vi "Debug Get Connected Units.vi"() -> ()   [LabVIEW 2021]
uses:
  <vilib>/Utility/config.llb/NI_LVConfig.lvlib
  <vilib>/Utility/config.llb/Read Key (Boolean).vi
panel:
  out "Array":T1(array[cluster])
  in  "stop":bool
  in  "UDP Config Publish Port":u16
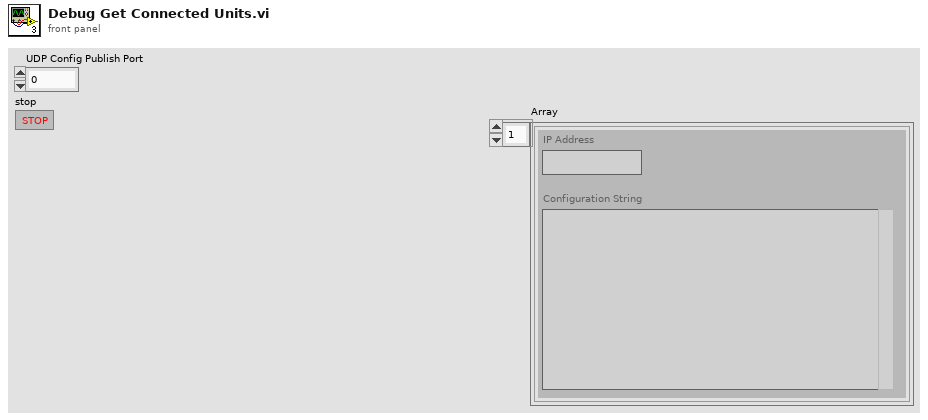
[diagram p1: front panel]
types:
  T1 = cluster{"IP Address":string, "Configuration String":string}[]
  T2 = cluster{"IP Address":string, "Configuration String":string}
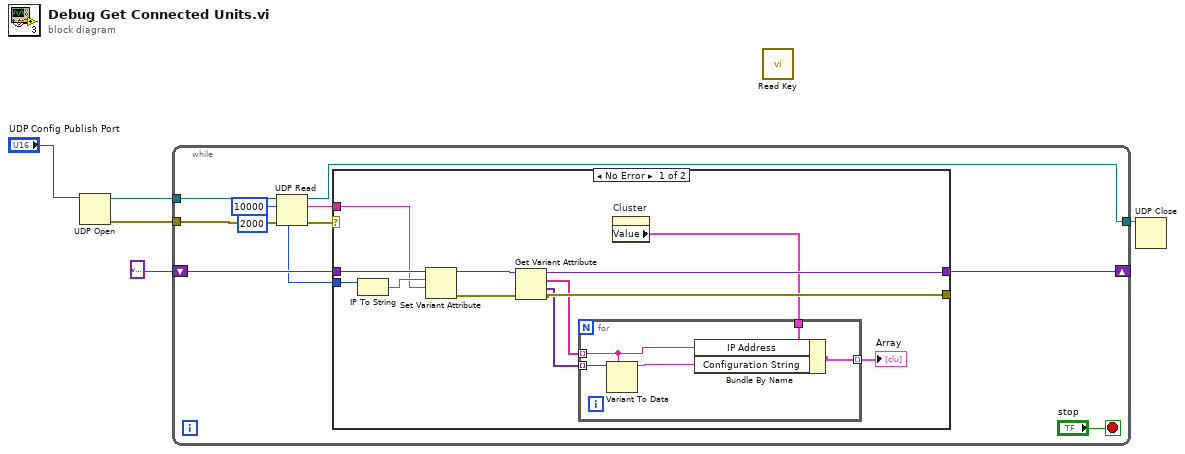
[diagram p0: block diagram]
diagram:
  n1 = UDP Open(11:"UDP Config Publish Port") -> (port=w3:refnum<k16>, 0:w4:errorcluster)  [unwired: 4 in, 1 out]
  n2 = while {
    tunnel: w4 -> [w16]
    tunnel: w3 -> [w15]
    shift-right: [w9] -> _
    shift-left: variant -> [w13]
    tunnel: [w7] -> w1
    stop <- "stop" stop-if-true
    n3 = UDP Read(connection ID=w15, max size (548)=10000, timeout ms (25000)=2000, 8:w16) -> (data out=w12:string, error out=w11:errorcluster, 3:w7:refnum<k16>, 6:w6:u32)  [unwired: 1 out]
    n4 = case shown="No Error" w11 {
      tunnel: w13 -> [w28 w34]
      tunnel: w6 -> [w26 _]
      tunnel: w12 -> [w25 _]
      tunnel: [w23 w34] -> w9
      tunnel: [w21 _] -> _
      frame No Error {
        n5 = IP To String(2:w26) -> (0:w27:string)  [unwired: 1 in]
        n6 = Set Variant Attribute(Variant=w28, name=w27, value=w25) -> (Variant out=w24:variant, error out=w22:errorcluster)  [unwired: 1 in, 1 out]
        n7 = Get Variant Attribute(Variant=w24, error in=w22) -> (duplicate Variant=w23:variant, names=w20:string[], values=w19:variant[], error out=w21:errorcluster)  [unwired: 2 in]
        n8 = property on="Cluster" class="Clust (strict)"() -> ("Value"=w18:T2)  [unwired: 2 in, 2 out]
        n9 = for {
          tunnel: w20 -> [w31] mode=indexing
          tunnel: w19 -> [w33] mode=indexing
          tunnel: w18 -> [w32]
          tunnel: [w29] -> w17 mode=indexing
          n10 = Variant To Data(type=w31, Variant=w33) -> (data=w30:string)  [unwired: 1 in, 1 out]
          n11 = Bundle By Name(cluster=w32, "IP Address"=w31, "Configuration String"=w30) -> (w29:T2)
        }
        "Array" <- w17
      }
      frame Error {
        # "probably timeout"
      }
    }
  }
  n12 = call-poly <vilib>:"Read Key.vi"() -> ()  [unwired: 8 in, 4 out]
  n13 = UDP Close(connection ID=w1) -> ()  [unwired: 1 in, 2 out]
